vi "Read Lock.vi"(9 "Knob in":refnum<class "Knob.lvclass">) -> (3 "Knob out":refnum<class "Knob.lvclass">, 4 "Lock":bool)   [LabVIEW 2014, in "Knob.lvclass"]
uses:
  Knob.lvclass
  Knob.lvclass/Knob.ctl
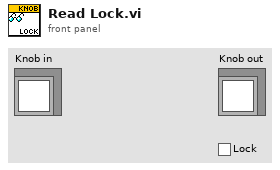
[diagram p1: front panel]
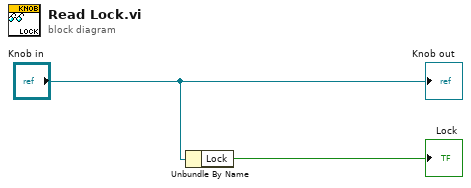
[diagram p0: block diagram]
diagram:
  n1 = Unbundle By Name("Knob in") -> ("Lock"=→"Lock":bool)
  "Knob out" <- "Knob in"
